vi "Launch PIMHW Engine.vi"(4 "Allow Connection with errors? (F)":bool, 6 "SIM OPTIONS":T1, 7 "Legacy (f)?":bool, 8 "error in (no error)":errorcluster, 9 "Force Simulation\n(ID = 0 gives no Sim)":u32, 10 "port (80)":u16=80, 11 "host (localhost)":string="localhost") -> (0 "error out":errorcluster, 3 "TestSetDef":T2={"General"={"ID"=0, "Model"="", "Dual Port?"=FALSE, "Options"="", "Options"={"E"=FALSE, "K"=FALSE, "H"=FALSE, "W"=FALSE, "F"=FALSE}, "Cal File"=path ""}, "Receiver"={"Fstart, MHz"=0.0, "Fstop MHz"=0.0, "Fstep MHz"=0.0, "IF, MHz"=0.0}, "RX Band"={"Fstart, MHz"=0.0, "Fstop MHz"=0.0}, "TX 1"={"Fstart, MHz"=0.0, "Fstop MHz"=0.0, "Pmax, dBm"=0.0, "Pstep, dB"=0.0}, "TX 2"={"Fstart, MHz"=0.0, "Fstop MHz"=0.0, "Pmax, dBm"=0.0, "Pstep, dB"=0.0}, "Low-side?"=TRUE}, 5 "Connection Ref":refnum<k5>)   [LabVIEW 2011]
doc: "Connects to the PIM hardware engine (pimhw.exe). The server must be running and not already connected. Successful connection causes the server to fire up the HWProcLoop and returns \"READY\" on TCP. Unresolved errors will force the connection closed by this VI.\n\nAfter successful connection, the hardware may be forced to \"simulation\" by entering a valid test set id. Leaving the default ID (0) will not force simulation.\n\nThe Test Set Definition is returned for successful connection for either simulated or actual hardware running under the server."
uses:
  HW IO/Test Set Definition.ctl
  HW IO/HWIO Global.vi
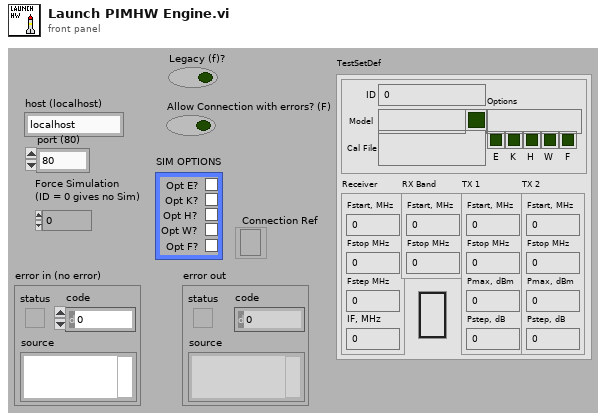
[diagram p1: front panel]
types:
  T1 = cluster{"Opt E?":bool, "Opt K?":bool, "Opt H?":bool, "Opt W?":bool, "Opt F?":bool}
  T2 = typedef "Test Set Definition.ctl" = cluster{"General":cluster{"ID":u32, "Model":string, "Dual Port?":bool, "Options":string, "Options":cluster{"E":bool, "K":bool, "H":bool, "W":bool, "F":bool}, "Cal File":path}, "Receiver":cluster{"Fstart, MHz":dbl, "Fstop MHz":dbl, "Fstep MHz":dbl, "IF, MHz":dbl}, "RX Band":cluster{"Fstart, MHz":dbl, "Fstop MHz":dbl}, "TX 1":cluster{"Fstart, MHz":dbl, "Fstop MHz":dbl, "Pmax, dBm":dbl, "Pstep, dB":dbl}, "TX 2":cluster{"Fstart, MHz":dbl, "Fstop MHz":dbl, "Pmax, dBm":dbl, "Pstep, dB":dbl}, "Low-side?":bool}
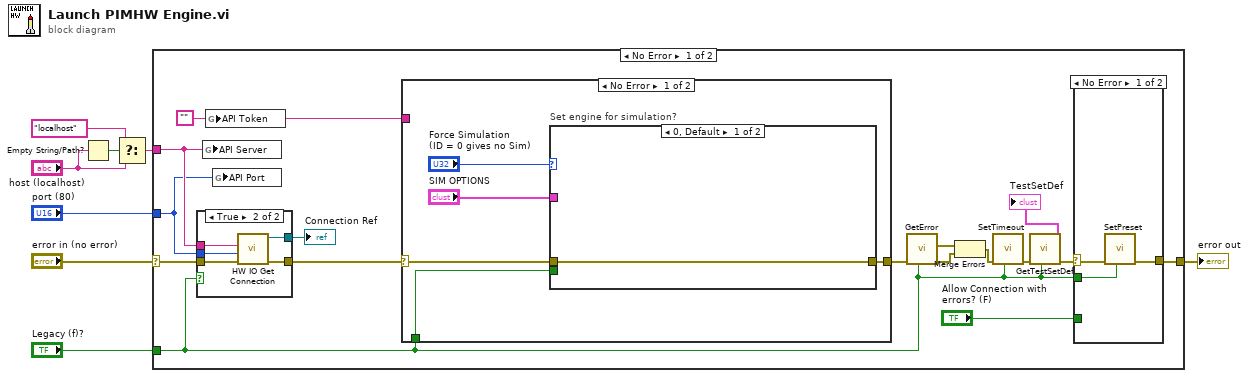
[diagram p0: block diagram]
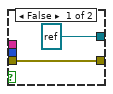
[diagram p2: hidden frame]
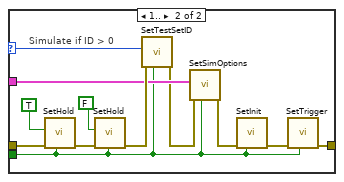
[diagram p3: hidden frame]
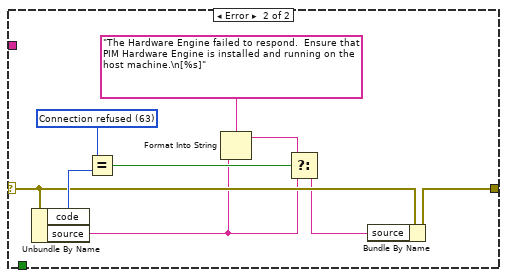
[diagram p4: hidden frame]
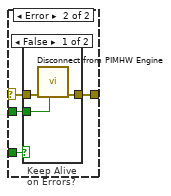
[diagram p5: hidden frame]
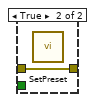
[diagram p6: hidden frame]
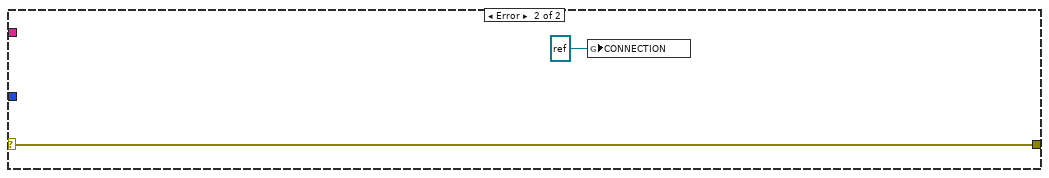
[diagram p7: hidden frame]
diagram:
  n1 = Empty String/Path?(string/path="host (localhost)") -> (empty?=w4:bool)
  n2 = Select(t="localhost" ("address"), s=w4, f="host (localhost)") -> (s? t:f=w2:string)
  n3 = case shown="No Error" "error in (no error)" {
    selector: "error in (no error)" -> [w16 w71]
    tunnel: [w23 w71] -> w8
    tunnel: "port (80)" -> [w13 _]
    tunnel: w2 -> [w14 _]
    tunnel: "Legacy (f)?" -> [w10 _]
    frame No Error {
      w9 = ""
      n4 = case shown="True" w10 {
        tunnel: [w25 w31] -> w21
        tunnel: w13 -> [_ w30]
        tunnel: w14 -> [_ w29]
        tunnel: w16 -> [w25 w28]
        tunnel: [refnum<k5> refnum ("connection ID") w27] -> w15
        frame False {
        }
        frame True {
          n5 = call "HW IO Get Connection.vi"("error in (no error)"=w28, "Port"=w30, "Server"=w29) -> ("error out"=w31:errorcluster, "connection ID"=w27:refnum<k5>)  [unwired: 5 in, 2 out]
        }
      }
      "Connection Ref" <- w15
      n6 = global write "HWIO Global.vi" "API Server"(w14) -> ()
      n7 = global write "HWIO Global.vi" "API Token"(w9) -> ()
      n8 = global write "HWIO Global.vi" "API Port"(w13) -> ()
      n9 = case shown="No Error" w21 {
        selector: w21 -> [w35 w55]
        tunnel: [w32 w53] -> w18
        tunnel: w10 -> [w33 _]
        tunnel: w9 -> [_ _]
        frame No Error {
          n10 = case "Set engine for simulation?" shown="0, Default" "Force Simulation\n(ID = 0 gives no Sim)" {
            selector: "Force Simulation\n(ID = 0 gives no Sim)" -> [_ w39]
            tunnel: [w37 w44] -> w32
            tunnel: w35 -> [w37 w43]
            tunnel: "SIM OPTIONS" -> [_ w42]
            tunnel: w33 -> [_ w38]
            frame 0, Default {
            }
            frame 1.. {
              # "Simulate if ID > 0"
              n11 = call "SetHold.vi"("Legacy (f)?"=w38, "error in (no error)"=w43, "Hold"=TRUE) -> ("error out"=w49:errorcluster)  [unwired: 8 out]
              n12 = call "SetHold.vi"("Legacy (f)?"=w38, "error in (no error)"=w49, "Hold"=FALSE) -> ("error out"=w48:errorcluster)  [unwired: 8 out]
              n13 = call "SetTestSetID.vi"("Legacy (f)?"=w38, "error in (no error)"=w48, "TestSetID"=w39) -> ("error out"=w41:errorcluster)  [unwired: 8 out]
              n14 = call "SetSimOptions.vi"("Legacy (f)?"=w38, "error in (no error)"=w41, "SIM OPTIONS"=w42) -> ("error out"=w40:errorcluster)  [unwired: 8 out]
              n15 = call "SetInit.vi"("Legacy (f)?"=w38, "error in (no error)"=w40) -> ("error out"=w45:errorcluster)  [unwired: 9 out]
              n16 = call "SetTrigger.vi"("Legacy (f)?"=w38, "error in (no error)"=w45) -> ("error out"=w44:errorcluster)  [unwired: 9 out]
            }
          }
        }
        frame Error {
          w58 = 63 items=["No error", "Argument error", "Memory is full", "Out of zone", "End of file", "File already open", "Generic file I/O error", "File not found", "File permission error", "Disk is full", "Duplicate path", "Too many files open", "System feature not enabled", "Resource file not found", "Cannot add resource", "Resource not found", "Image not found", "Image memory error", "Pen does not exist", "Config type invalid", "Config token not found", "Config parse error", "Config memory error", "Bad external code format", "Bad external code offset", "External code not present", "Null window", "Destroy window error", "Null menu", "Print aborted", "Bad print record", "Print driver error", "Windows error during printing", "Memory error during printing", "Print dialog error", "Generic print error", "Invalid device refnum", "Device not found", "Device parameter error", "Device unit error", "Cannot open device", "Device call aborted", "Generic error", "Cancelled by user", "Object ID too low", "Object ID too high", "Object not in heap", "Unknown heap", "Unknown object (invalid DefProc)", "Unknown object (DefProc not in table)", "Message out of range", "Invalid (null) method", "Unknown message", "Manager call not supported", "Bad address", "Network operation in progress", "Network operation timed out", "Connection is busy", "Network attribute not supported", "Network error", "Address in use", "System out of memory", "Connection aborted", "Connection refused", "Not connected", "Already connected", "Connection closed", "Initialization error (interapplication manager)", "Bad occurrence", "Wait on unbound occurrence handler", "Occurrence queue overflow", "Datalog type conflict", "Unused", "Unrecognized type (interapplication manager)", "Memory corrupt", "Failed to make temporary DLL", "Old CIN version", "Drag socket not found", "Failed to load drop-object", "Failed to register OLE object", "Failed to release OLE object", "Format specifier type mismatch", "Unknown format specifier", "Too few format specifiers", "Too many format specifiers", "Scan failed", "Newer CIN version", "Error converting to variant", "Runtime menu error", "Password tampered", "Variant attribute not found", "Incompatible variant data type", "Event data is not available", "Event Store is not present", "Occurrence is not found", "Event Queue is not created", "Event info is not available in the type library", "Refnum passed is NULL", "Error retrieving Class GUID", "Error retrieving CoClass GUID", "Error retrieving TypeLib GUID.", "Bad built application magic bytes.", "Specific driver is different from the specific driver associated with the Logical Name.", "There is no session opened to the class driver.", "Max Error", "MAX - Error with config objects", "MAX - Error loading configuration", "MAX - Group not supported", "Singlecast connections can not send to multicast addresses.", "Multicast connections can not send to singlecast addresses.", "Specified IP address not in multicast address range.", "Attempt to write to read-only multicast connection.", "Attempt to read from write-only multicast connection.", "The buffer used to receive a datagram was smaller than the datagram itself"] ("x")
          n17 = Unbundle By Name(w55) -> ("code"=w57:i32, "source"=w51:string)
          n18 = Equal?(x=w58, y=w57) -> (x = y?=w56:bool)
          n19 = Format Into String(format string="The Hardware Engine failed to respond.  Ensure that PIM Hardware Engine is installed and running on the host machine.\n[%s]" ("source"), w51) -> (resulting string=w50:string)  [unwired: 2 in, 1 out]
          n20 = Select(t=w50, s=w56, f=w51) -> (s? t:f=w54:string)
          n21 = Bundle By Name(cluster=w55, "source"=w54) -> (w53:errorcluster)
        }
      }
      n22 = call "GetError.vi"("Legacy (f)?"=w10, "error in (no error)"=w18) -> ("error out"=w19:errorcluster, "HW Error"=w20:errorcluster)  [unwired: 8 out]
      n23 = Merge Errors(w20, w19) -> (w12:errorcluster)
      n24 = call "SetTimeout.vi"("Legacy?"=w10, "error in (no error)"=w12) -> ("error out"=w11:errorcluster)  [unwired: 9 in]
      n25 = call "GetTestSetDef.vi"("Legacy (f)?"=w10, "error in (no error)"=w11) -> ("error out"=w24:errorcluster, "TestSetDef"=→"TestSetDef":T2)  [unwired: 8 out]
      n26 = case shown="No Error" w24 {
        selector: w24 -> [w61 w65]
        tunnel: [w60 w64] -> w23
        tunnel: "Allow Connection with errors? (F)" -> [_ w63]
        tunnel: w10 -> [w59 w62]
        frame No Error {
          n27 = call "SetPreset.vi"("Legacy (f)?"=w59, "error in (no error)"=w61) -> ("error out"=w60:errorcluster)  [unwired: 9 in]
        }
        frame Error {
          n28 = case "Keep Alive\non Errors?" shown="False" w63 {
            tunnel: w65 -> [w68 w69]
            tunnel: [w67 w69] -> w64
            tunnel: w62 -> [w66 _]
            frame False {
              n29 = call "Disconnect from PIMHW Engine.vi"("Legacy (f)?"=w66, "error in (no error)"=w68) -> ("error out"=w67:errorcluster)  [unwired: 9 in]
            }
            frame True {
              n30 = call "SetPreset.vi"() -> ()  [unwired: 11 in, 1 out]
            }
          }
        }
      }
    }
    frame Error {
      n31 = global write "HWIO Global.vi" "CONNECTION"(refnum<k5> refnum ("connection ID")) -> ()
    }
  }
  "error out" <- w8
